vi "Configure Analog Filter.vi"(0 "VISA resource name":refnum<visa-resource-name>, 1 "Measurement (0: Voltage Channel 1)":i32(ring) items=["Voltage Channel 1", "Voltage Channel 2", "Temperature Channel 1", "Temperature Channel 2"], 5 "Enable Analog Filter (T: Enable)":bool=TRUE, 11 "error in (no error)":errorcluster) -> (4 "VISA resource name out":refnum<visa-resource-name>, 15 "error out":errorcluster)   [LabVIEW 2019, in "Keithley 2182.lvlib"]
doc: "Configures analog filter settings for the selected measurement.\n\nWith the low-pass Analog Filter ON, the normal-mode noise rejection ratio of the instrument is increased at 60Hz. This filters out noise induced by the power line. The Analog Filter attenuates frequency at 20dB/decade starting at 18Hz.\n\nA primary use of the Analog Filter is to keep the high-gain input stage of the Model 2182 from saturating due to the presence of high AC and DC voltage. Note, however, that the filter only attenuates AC voltages for the 10mV range of the Model 2182.\n\nThe Analog Filter adds approximately 125msec of settling between A/D conversions. The additional settling time may be required when using a high-impedance ( > or = 100k ohms) source in the test circuit.\n\nThe increased settling time causes the reading rate of the Model 2182 to be greatly reduced. Therefore, if the Analog Filter is not needed, turn it OFF."
uses:
  Keithley 2182.lvlib
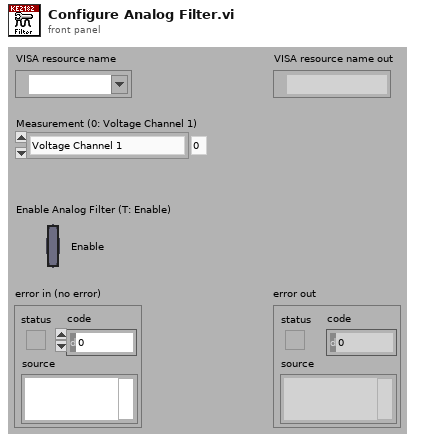
[diagram p1: front panel]
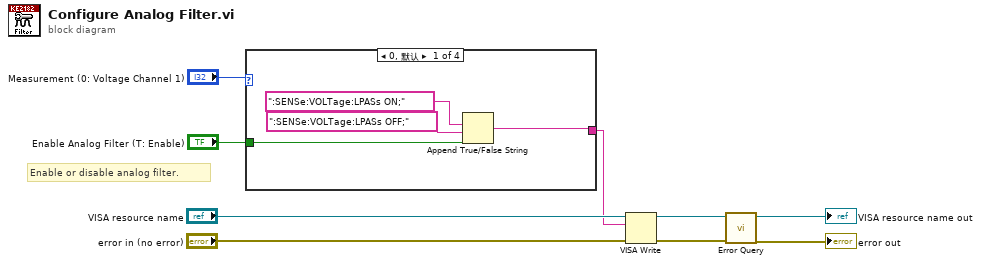
[diagram p0: block diagram]
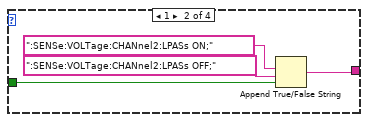
[diagram p2: hidden frame]
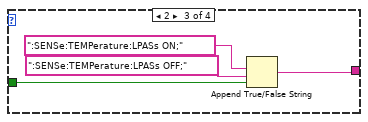
[diagram p3: hidden frame]
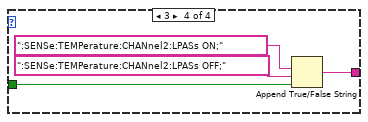
[diagram p4: hidden frame]
diagram:
  # "Enable or disable analog filter."
  n1 = case shown="0, 默认" "Measurement (0: Voltage Channel 1)" {
    tunnel: "Enable Analog Filter (T: Enable)" -> [w13 w15 w19 w23]
    tunnel: [w10 w14 w18 w22] -> w1
    frame 0, Default {
      n2 = Append True/False String(1:w13, 2:":SENSe:VOLTage:LPASs OFF;", 3:":SENSe:VOLTage:LPASs ON;") -> (0:w10:string)  [unwired: 1 in]
    }
    frame 1 {
      n3 = Append True/False String(1:w15, 2:":SENSe:VOLTage:CHANnel2:LPASs OFF;", 3:":SENSe:VOLTage:CHANnel2:LPASs ON;") -> (0:w14:string)  [unwired: 1 in]
    }
    frame 2 {
      n4 = Append True/False String(1:w19, 2:":SENSe:TEMPerature:LPASs OFF;", 3:":SENSe:TEMPerature:LPASs ON;") -> (0:w18:string)  [unwired: 1 in]
    }
    frame 3 {
      n5 = Append True/False String(1:w23, 2:":SENSe:TEMPerature:CHANnel2:LPASs OFF;", 3:":SENSe:TEMPerature:CHANnel2:LPASs ON;") -> (0:w22:string)  [unwired: 1 in]
    }
  }
  n6 = VISA Write(VISA resource name="VISA resource name", write buffer=w1, error in (no error)="error in (no error)") -> (VISA resource name out=w6:refnum<visa-resource-name>, error out=w5:errorcluster)  [unwired: 1 out]
  n7 = call "Error Query.vi"("error in (no error)"=w5, "VISA resource name"=w6) -> ("error out"=→"error out":errorcluster, "VISA resource name out"=→"VISA resource name out":refnum<visa-resource-name>)  [unwired: 6 in, 2 out]
